vi "Set Intensity Scales (array).vi"(7 "IntensityGraph in":refnum<vi>, 8 "error in (no error)":errorcluster, 9 "Y Scale":dbl[](array[numeric]), 10 "X Scale":dbl[](array[numeric]), 11 "Intensity Data":dbl[][](array[numeric])) -> (0 "error out":errorcluster)   [LabVIEW 2016, in "graph_utilities.lvlib"]
uses:
  graph_utilities.lvlib
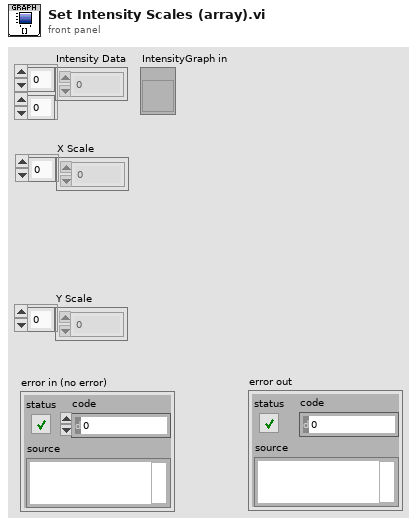
[diagram p1: front panel]
types:
  T1 = typedef "LVOffsetAndMultiplierTypeDef.ctl" = cluster{"Offset":dbl, "Multiplier":dbl}
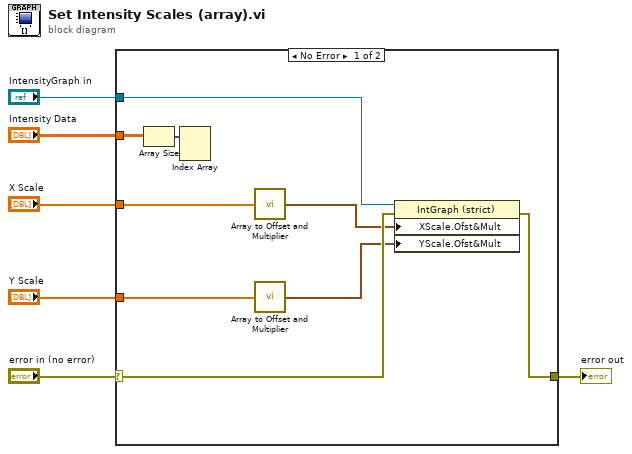
[diagram p0: block diagram]
diagram:
  n1 = case shown="No Error" "error in (no error)" {
    selector: "error in (no error)" -> [w11 w16]
    tunnel: "Intensity Data" -> [w14 _]
    tunnel: "Y Scale" -> [w9 _]
    tunnel: "X Scale" -> [w10 _]
    tunnel: [w13 w16] -> w3
    tunnel: "IntensityGraph in" -> [w12 _]
    frame No Error {
      n2 = Array Size(array=w14) -> (size(s)=w15:i32[])
      n3 = Index Array(array=w15) -> ()  [unwired: 2 in, 2 out]
      n4 = call "Array to Offset and Multiplier.vi"("Array"=w10) -> ("Offset and Multiplier"=w7:T1)
      n5 = call "Array to Offset and Multiplier.vi"("Array"=w9) -> ("Offset and Multiplier"=w8:T1)
      n6 = property on="Property Node" class="IntGraph (strict)"(reference=w12, error in=w11, "XScale.Ofst&Mult"=w7, "YScale.Ofst&Mult"=w8) -> (error out=w13:errorcluster)  [unwired: 1 out]
    }
    frame Error {
    }
  }
  "error out" <- w3
